vi "Parse YAML.vi"() -> ()   [LabVIEW 2020]
uses:
  <vilib>/regexp/Match Regular Expression.xnode
panel:
  in  "Rename":string[](array[string])
  in  "Original":string[](array[string])
  out "Array 3":i32[](array[numeric])=[0, 6, 1, 3]
  in  "Load Notes":bool
  out "B":u16(ring)=3 items=["OFF", "Magnet Field", "Temperature", "Magnet", "Time", "Vsg", "X1", "Y1", "X2", "Y2", "X3", "Y3", "X4", "Y4", "X5", "Y5", "X6", "Y6", "X7", "Y7", "X8", "Y8"]
  out "Vsg":u16(ring)=12 items=["OFF", "Magnet Field", "Temperature", "Magnet", "Time", "Vsg", "X1", "Y1", "X2", "Y2", "X3", "Y3", "X4", "Y4", "X5", "Y5", "X6", "Y6", "X7", "Y7", "X8", "Y8"]
  out "CURRENT":u16(ring)=8 items=["OFF", "Magnet Field", "Temperature", "Magnet", "Time", "Vsg", "X1", "Y1", "X2", "Y2", "X3", "Y3", "X4", "Y4", "X5", "Y5", "X6", "Y6", "X7", "Y7", "X8", "Y8"]
  out "V2":u16(ring)=18 items=["OFF", "Magnet Field", "Temperature", "Magnet", "Time", "Vsg", "X1", "Y1", "X2", "Y2", "X3", "Y3", "X4", "Y4", "X5", "Y5", "X6", "Y6", "X7", "Y7", "X8", "Y8"]
  in  "Read TDMS Data":bool=TRUE
  in  "TDMS Path":path=path "G:/My Drive/ansom/Data/PPMSDAQ/2020/PPMS 1/SA02821O.20201219/03-Sweep B Vsg lockin/SA02821O.20201219.000000.tdms"
  in  "Load Wavenames":bool
  out "V1":u16(ring)=6 items=["OFF", "Magnet Field", "Temperature", "Magnet", "Time", "Vsg", "X1", "Y1", "X2", "Y2", "X3", "Y3", "X4", "Y4", "X5", "Y5", "X6", "Y6", "X7", "Y7", "X8", "Y8"]
  out "Array":string[](array[string])=["V1-", "I-", "", "Vsg", "", "", "V1+", "I+"]
  in  "# Channels":i32=8
  in  "format string":string="Lockin %d, "
  in  "Notes":string="Device: \r  Device Name: SA02821O.20201219\r  Computer: PPMSDAQ\r  User: Muqing\r  Instrument: PPMS 1\r  Description: |\r\rExperiment: \r  Time: 2020-12-19T23:12:41\r  Description: |\r    B sweep from -9T to 9T, 0.2T step\r    Vsg sweep from -10 mV to 210 mV 300s\r    T < 90 mK\r    Vbg = -0.5 V\r    \r    I+/-: 28/2 0.15 mV ac + -300 uV dc, 13 Hz\r    V1+/-: 27/1 \r    \r    tc = 250 ms\r    filter: on\r\rSweep: \r- Loop1: [Magnet Field, -9.000000]\r- Loop2: [OFF, 0.000000]\r- Loop3: [OFF, 0.200000]\r- Loop4: [OFF, 0.000000]\r\rWiring: \r- Electrode 1: Lockin 1, V1-, KH1 Channel 1, SE+ (-gnd), 10x, Open\r- Electrode 2: Lockin 2, I-, KH1 Channel 2, Differential, 10x, 50k Ohms\r- Electrode 3: Lockin 3, , KH1 Channel 3, Ground, 10x, Open\r- Electrode 4: Lockin 4, Vsg, KH1 Channel 4, Differential, 10x, 50k Ohms\r- Electrode 5: Lockin 5, , KH1 Channel 5, Ground, 10x, Open\r- Electrode 6: Lockin 6, , KH1 Channel 6, Ground, 10x, Open\r- Electrode 7: Lockin 7, V1+, KH1 Channel 7, SE+ (-gnd), 10x, Open\r- Electrode 8: Lockin 8, I+, KH1 Channel 8, Differential, 10x, 50k Ohms\r\rLockin: \r  AO: \r  - AO 1: amp = 0.000 mV, DC = 0.000 mV, f = 13.00 Hz, phi = 0.00°, Triangle\r  - AO 2: amp = 0.000 mV, DC = 0.000 mV, f = 13.00 Hz, phi = 0.00°, Triangle\r  - AO 3: amp = 0.000 mV, DC = 0.000 mV, f = 13.00 Hz, phi = 0.00°, Sine\r  - AO 4: amp = 0.000 mV, DC = -10.000 mV, f = 13.00 Hz, phi = 0.00°, Sine\r  - AO 5: amp = 0.000 mV, DC = 0.000 mV, f = 13.00 Hz, phi = 0.00°, Sine\r  - AO 6: amp = 0.000 mV, DC = 0.000 mV, f = 13.00 Hz, phi = 0.00°, Sine\r  - AO 7: amp = 0.000 mV, DC = 0.000 mV, f = 13.00 Hz, phi = 0.00°, Sine\r  - AO 8: amp = 0.150 mV, DC = -0.300 mV, f = 13.00 Hz, phi = 0.00°, Triangle\r  REF: \r  - Lockin 1: f = 13.00 Hz, phi = 0.00°, TC = 0.25 s, order = 2 \r  Sampling: \r  - Fs: 195000.000000\r  - N: 15000\r"
  # "Configure Read TDMS File"
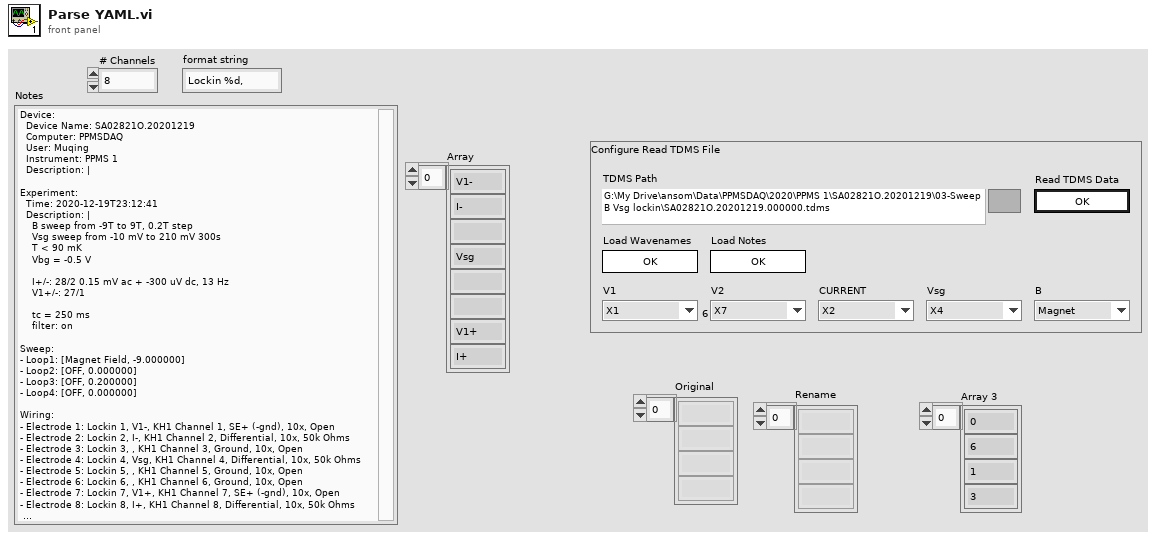
[diagram p1: front panel]
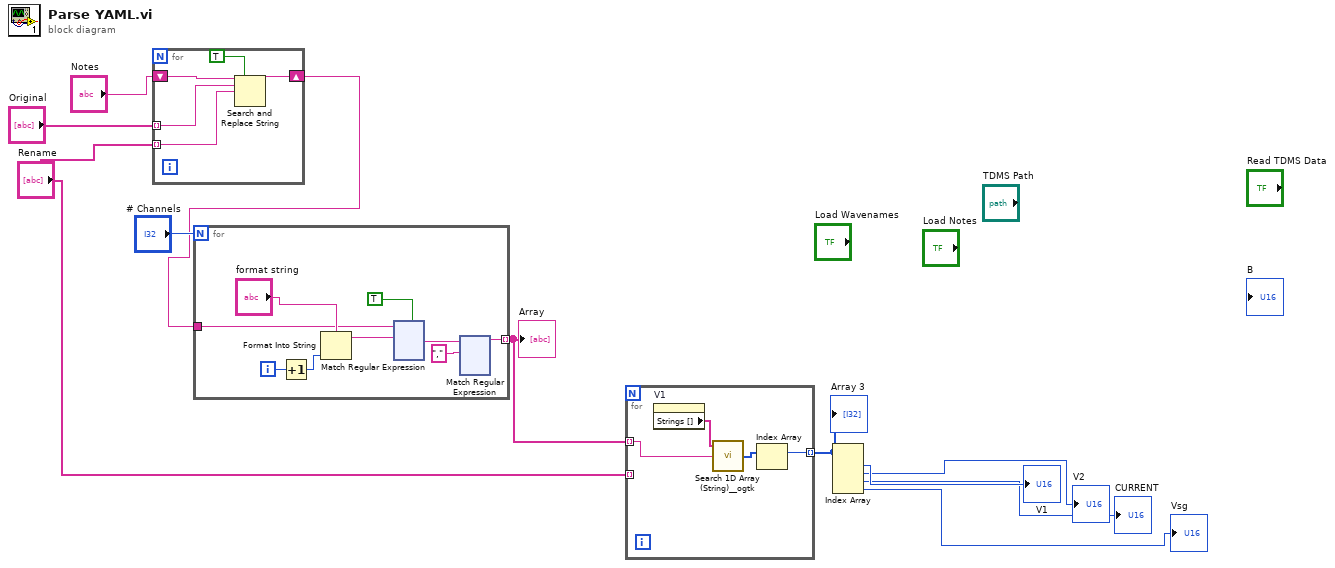
[diagram p0: block diagram]
diagram:
  n1 = for {
    shift-right: [w16] -> w8
    shift-left: "Notes" -> [w15]
    tunnel: "Original" -> [w13] mode=indexing
    tunnel: "Rename" -> [w12] mode=indexing
    n2 = Search and Replace String(replace all?=TRUE ("replace all? (F)"), input string=w15, search string=w13, replace string=w12) -> (result string=w16:string)  [unwired: 4 in, 3 out]
  }
  n3 = for {
    N: "# Channels" -> [_]
    tunnel: [w24] -> w10 mode=indexing
    tunnel: w8 -> [w17]
    i -> [w21]
    n4 = Increment(x=w21) -> (x+1=w20:i32)
    n5 = Format Into String(format string="format string", w20) -> (resulting string=w18:string)  [unwired: 2 in, 1 out]
    n6 = xnode "Match Regular Expression"("input string"=w17, "regular expression"=w18, "multiline? (F)"=TRUE) -> ("after match"=w22:string)  [unwired: 3 in, 4 out]
    n7 = xnode "Match Regular Expression"("input string"=w22, "regular expression"=",") -> ("before match"=w24:string)  [unwired: 4 in, 4 out]
  }
  "Array" <- w10
  n8 = for {
    tunnel: w10 -> [w256] mode=indexing
    tunnel: "Rename" -> [_] mode=indexing
    tunnel: [w254] -> w1 mode=indexing
    n9 = property on="V1" class="Ring (strict)"() -> ("Strings []"=w257:string[])  [unwired: 2 in, 2 out]
    n10 = call <userlib>:"Search 1D Array (String)__ogtk.vi"("Array"=w257, "Element Data"=w256) -> ("Indices of Elements"=w255:i32[])  [unwired: 7 in]
    n11 = Index Array(array=w255) -> (element=w254:i32)  [unwired: 1 in]
  }
  "Array 3" <- w1
  n12 = Index Array(array=w1) -> (element #1=→"V1":i32, element #2=→"V2":i32, element #3=→"CURRENT":i32, element #4=→"Vsg":i32)  [unwired: 4 in]
